vi "fluorescence_timing_pb.vi"(1 "Less frequently changed controls":T2={"Column for Fluorescence"=11, "PB Ch for Blue Image AOM"=5, "PB Ch for Blue MOT AOM"=6, "PB Ch for MOT Shutter"=7, "MOT Shutter Open Time (s)"=0.05}, 2 "Fluorescence Control":T1={"Absorption or Fluorescence?"=0, "MOT flash time (us)"=500.0} {"Absorption or Fluorescence?" items=["Absorption", "Fluorescence"]}, 3 "PulseBlaster Array of Arrays In":T3(array[cluster])=[{"Data Field"=0, "Delay"=0.005, "OP code"=8, "Output Bits"=[FALSE, TRUE, FALSE, FALSE, FALSE, TRUE, FALSE, FALSE, FALSE, FALSE, FALSE, FALSE, FALSE, FALSE, FALSE, FALSE, FALSE, FALSE, FALSE, FALSE, FALSE, FALSE, FALSE, FALSE], "String"="cool mot coils"}, {"Data Field"=300, "Delay"=0.000999, "OP code"=2, "Output Bits"=[FALSE, TRUE, FALSE, FALSE, FALSE, TRUE, FALSE, FALSE, FALSE, FALSE, FALSE, FALSE, FALSE, FALSE, FALSE, FALSE, FALSE, FALSE, FALSE, FALSE, FALSE, FALSE, FALSE, FALSE], "String"="mot load loop"}, {"Data Field"=1, "Delay"=1e-06, "OP code"=3, "Output Bits"=[FALSE, TRUE, FALSE, FALSE, FALSE, TRUE, FALSE, FALSE, FALSE, FALSE, FALSE, FALSE, FALSE, FALSE, FALSE, FALSE, FALSE, FALSE, FALSE, FALSE, FALSE, FALSE, FALSE, FALSE, FALSE], "String"=""}, {"Data Field"=0, "Delay"=0.001, "OP code"=0, "Output Bits"=[FALSE, TRUE, FALSE, FALSE, FALSE, TRUE, TRUE, FALSE, FALSE, FALSE, FALSE, FALSE, FALSE, FALSE, FALSE, FALSE, FALSE, FALSE, FALSE, FALSE, FALSE, FALSE, FALSE, FALSE], "String"=""}, {"Data Field"=2, "Delay"=0.000999, "OP code"=2, "Output Bits"=[FALSE, TRUE, FALSE, FALSE, FALSE, TRUE, TRUE, FALSE, FALSE, FALSE, FALSE, FALSE, FALSE, FALSE, FALSE, FALSE, FALSE, FALSE, FALSE, FALSE, FALSE, FALSE, FALSE, FALSE], "String"="mot decay loop"}, {"Data Field"=4, "Delay"=1e-06, "OP code"=3, "Output Bits"=[FALSE, TRUE, FALSE, FALSE, FALSE, TRUE, TRUE, FALSE, FALSE, FALSE, FALSE, FALSE, FALSE, FALSE, FALSE, FALSE, FALSE, FALSE, FALSE, FALSE, FALSE, FALSE, FALSE, FALSE], "String"=""}, {"Data Field"=0, "Delay"=0.04, "OP code"=0, "Output Bits"=[FALSE, TRUE, FALSE, FALSE, FALSE, TRUE, TRUE, FALSE, FALSE, FALSE, FALSE, FALSE, FALSE, FALSE, FALSE, FALSE, FALSE, FALSE, FALSE, FALSE, FALSE, FALSE, FALSE, FALSE], "String"=""}, {"Data Field"=0, "Delay"=0.00865, "OP code"=0, "Output Bits"=[FALSE, TRUE, FALSE, FALSE, FALSE, FALSE, TRUE, FALSE, FALSE, FALSE, FALSE, FALSE, FALSE, FALSE, FALSE, FALSE, FALSE, FALSE, FALSE, FALSE, FALSE, FALSE, FALSE, FALSE], "String"=""}, {"Data Field"=0, "Delay"=0.004, "OP code"=0, "Output Bits"=[FALSE, TRUE, FALSE, FALSE, FALSE, FALSE, TRUE, FALSE, FALSE, FALSE, FALSE, FALSE, FALSE, FALSE, FALSE, FALSE, FALSE, FALSE, FALSE, FALSE, FALSE, FALSE, FALSE, FALSE], "String"=""}, {"Data Field"=0, "Delay"=0.0045, "OP code"=0, "Output Bits"=[FALSE, TRUE, FALSE, FALSE, FALSE, FALSE, TRUE, FALSE, FALSE, FALSE, FALSE, FALSE, FALSE, FALSE, FALSE, FALSE, FALSE, FALSE, FALSE, FALSE, FALSE, FALSE, FALSE, FALSE], "String"="Blue MOT Cooling Time"}, {"Data Field"=0, "Delay"=5e-05, "OP code"=0, "Output Bits"=[FALSE, TRUE, FALSE, FALSE, FALSE, FALSE, TRUE, FALSE, FALSE, FALSE, FALSE, FALSE, FALSE, FALSE, FALSE, FALSE, FALSE, FALSE, FALSE, FALSE, FALSE, FALSE, FALSE, FALSE], "String"="Red MOT Cooling Time =="}, {"Data Field"=0, "Delay"=0.01, "OP code"=0, "Output Bits"=[FALSE, TRUE, FALSE, FALSE, FALSE, FALSE, TRUE, FALSE, FALSE, FALSE, FALSE, FALSE, FALSE, FALSE, FALSE, FALSE, FALSE, FALSE, FALSE, FALSE, FALSE, FALSE, FALSE, FALSE], "String"="PAS Beam with RED MOT            DELAY TIME BEFORE INTERAC"}, {"Data Field"=0, "Delay"=0.005, "OP code"=0, "Output Bits"=[FALSE, TRUE, FALSE, FALSE, TRUE, FALSE, TRUE, FALSE, FALSE, FALSE, FALSE, FALSE, FALSE, FALSE, FALSE, FALSE, FALSE, FALSE, FALSE, FALSE, FALSE, FALSE, FALSE, FALSE], "String"="image 12 delay (150n=90ndelay) INTERAC TIME"}, {"Data Field"=0, "Delay"=5e-05, "OP code"=0, "Output Bits"=[FALSE, TRUE, FALSE, FALSE, TRUE, FALSE, TRUE, FALSE, FALSE, FALSE, FALSE, FALSE, FALSE, FALSE, FALSE, FALSE, FALSE, FALSE, FALSE, FALSE, FALSE, FALSE, FALSE, FALSE], "String"="image beam on"}, {"Data Field"=0, "Delay"=0.0002, "OP code"=0, "Output Bits"=[FALSE, TRUE, FALSE, FALSE, FALSE, FALSE, TRUE, FALSE, FALSE, FALSE, FALSE, FALSE, FALSE, FALSE, FALSE, FALSE, FALSE, FALSE, FALSE, FALSE, FALSE, FALSE, FALSE, FALSE], "String"="camera minimum exposure time"}, {"Data Field"=0, "Delay"=0.07, "OP code"=0, "Output Bits"=[FALSE, TRUE, FALSE, FALSE, FALSE, FALSE, TRUE, FALSE, FALSE, FALSE, FALSE, FALSE, FALSE, FALSE, FALSE, FALSE, FALSE, FALSE, FALSE, FALSE, FALSE, FALSE, FALSE, FALSE], "String"="PixelFly Readout 1"}, {"Data Field"=0, "Delay"=0.005, "OP code"=0, "Output Bits"=[FALSE, TRUE, FALSE, FALSE, TRUE, FALSE, TRUE, FALSE, FALSE, FALSE, FALSE, FALSE, FALSE, FALSE, FALSE, FALSE, FALSE, FALSE, FALSE, FALSE, FALSE, FALSE, FALSE, FALSE], "String"="shutter opening time"}, {"Data Field"=0, "Delay"=0.0002, "OP code"=0, "Output Bits"=[FALSE, TRUE, FALSE, FALSE, FALSE, FALSE, TRUE, FALSE, FALSE, FALSE, FALSE, FALSE, FALSE, FALSE, FALSE, FALSE, FALSE, FALSE, FALSE, FALSE, FALSE, FALSE, FALSE, FALSE], "String"="Pixelfly exposure 2"}, {"Data Field"=0, "Delay"=0.07, "OP code"=0, "Output Bits"=[FALSE, TRUE, FALSE, FALSE, FALSE, FALSE, TRUE, FALSE, FALSE, FALSE, FALSE, FALSE, FALSE, FALSE, FALSE, FALSE, FALSE, FALSE, FALSE, FALSE, FALSE, FALSE, FALSE, FALSE], "String"="PixelFly readout 2"}, {"Data Field"=0, "Delay"=0.001, "OP code"=6, "Output Bits"=[FALSE, TRUE, FALSE, FALSE, FALSE, FALSE, TRUE, FALSE, FALSE, FALSE, FALSE, FALSE, FALSE, FALSE, FALSE, FALSE, FALSE, FALSE, FALSE, FALSE, FALSE, FALSE, FALSE, FALSE], "String"=""}] {"OP code" items=["Continue", "Stop", "Loop", "End Loop", "Jump", "Return", "Go To", "Long Delay", "Wait"]; "Delay" format="%.3p"}) -> (0 "PB Array of Arrays Out":T3(array[cluster]) {"OP code" items=["Continue", "Stop", "Loop", "End Loop", "Jump", "Return", "Go To", "Long Delay", "Wait"]; "Delay" format="%.2p"})   [LabVIEW 2013]
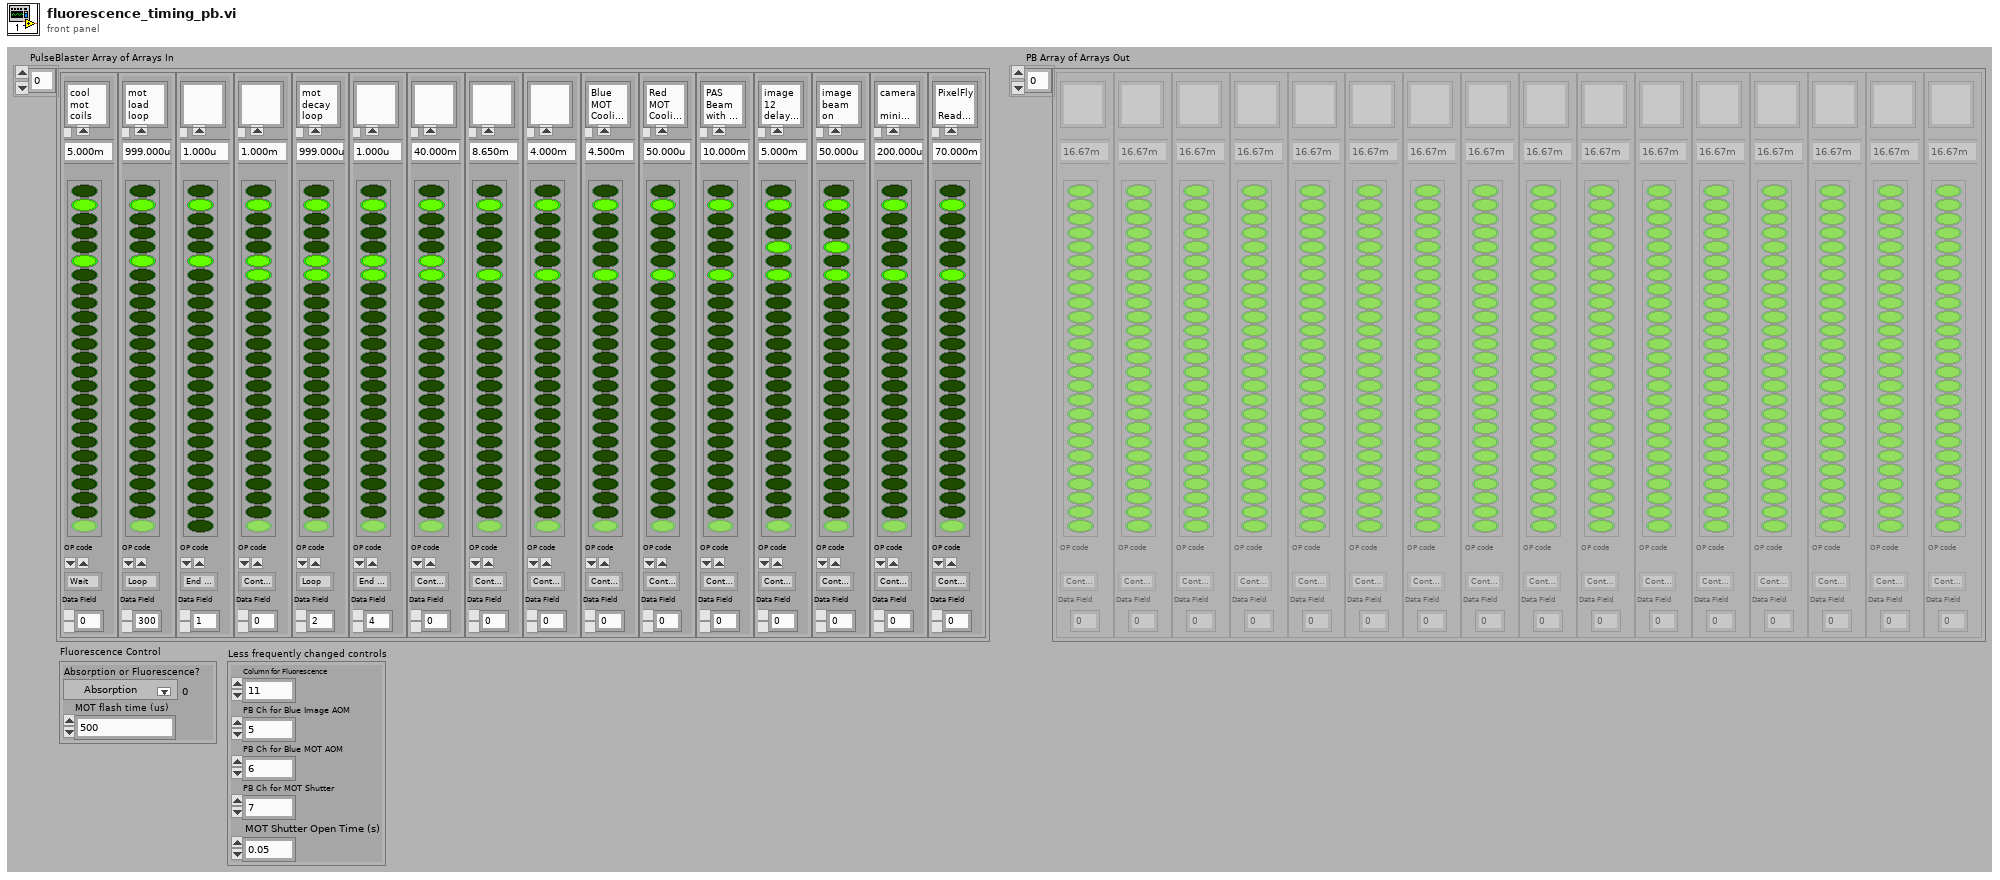
[diagram p1: front panel]
types:
  T1 = cluster{"Absorption or Fluorescence?":u16, "MOT flash time (us)":dbl}
  T2 = cluster{"Column for Fluorescence":i32, "PB Ch for Blue Image AOM":i32, "PB Ch for Blue MOT AOM":i32, "PB Ch for MOT Shutter":i32, "MOT Shutter Open Time (s)":dbl}
  T3 = cluster{"Data Field":u32, "Delay":dbl, "OP code":u8, "Output Bits":bool[], "String":string}[]
  T4 = cluster{"Data Field":u32, "Delay":dbl, "OP code":u8, "Output Bits":bool[], "String":string}
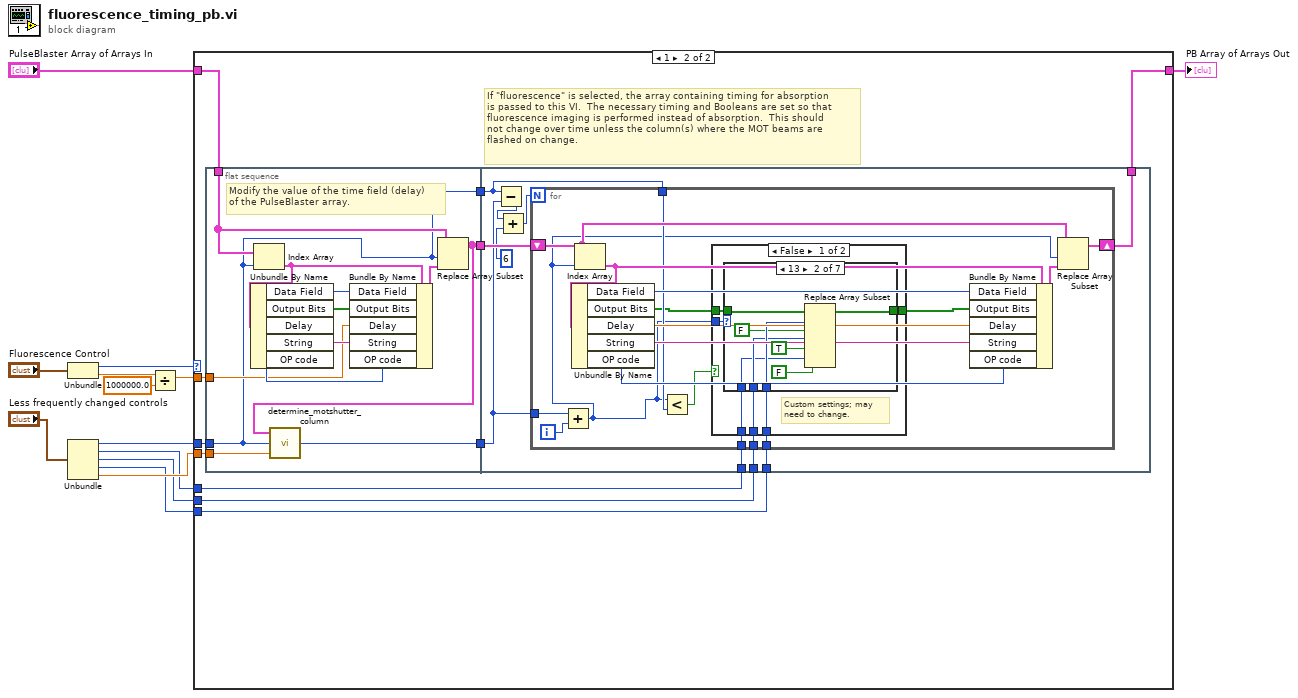
[diagram p0: block diagram]
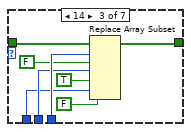
[diagram p4: hidden frame]
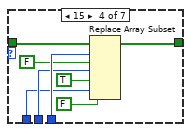
[diagram p5: hidden frame]
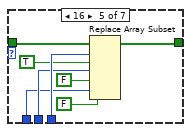
[diagram p6: hidden frame]
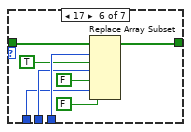
[diagram p7: hidden frame]
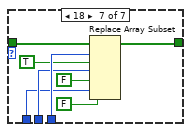
[diagram p8: hidden frame]
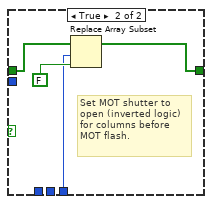
[diagram p9: hidden frame]
diagram:
  n1 = Unbundle("Fluorescence Control") -> ("Absorption or Fluorescence?"=w11:u16, "MOT flash time (us)"=w2:dbl)
  n2 = Unbundle("Less frequently changed controls") -> ("Column for Fluorescence"=w9:i32, "PB Ch for Blue Image AOM"=w6:i32, "PB Ch for Blue MOT AOM"=w5:i32, "PB Ch for MOT Shutter"=w4:i32, "MOT Shutter Open Time (s)"=w7:dbl)
  n3 = Divide(x=w2, y=1000000.0) -> (x/y=w3:dbl)
  n4 = case shown="1" w11 {
    tunnel: "PulseBlaster Array of Arrays In" -> [w14 w25]
    tunnel: w3 -> [_ w24]
    tunnel: w9 -> [_ w23]
    tunnel: [w14 w22] -> w8
    tunnel: w7 -> [_ w19]
    tunnel: w6 -> [_ w17]
    tunnel: w5 -> [_ w16]
    tunnel: w4 -> [_ w15]
    frame 0, Default {
      # "Default is absorption imaging.  The timing on the front panel\nof the PB stays just as it is."
    }
    frame 1 {
      # "If \"fluorescence\" is selected, the array containing timing for absorption\nis passed to this VI.  The necessary timing and Booleans are set so that\nfluorescence imaging is performed instead of absorption.  This should\nnot change over time unless the column(s) where the MOT beams are \nflashed on change."
      n5 = flat-sequence {
        tunnel: w25 -> [w31]
        tunnel: w24 -> [w30]
        tunnel: w23 -> [w26]
        tunnel: [w29] -> w21
        tunnel: [w27] -> w20
        tunnel: w19 -> [w28]
        tunnel: [w26] -> w18
        tunnel: w21 -> [w47]
        tunnel: w20 -> [w45]
        tunnel: [w46] -> w22
        tunnel: w18 -> [w41]
        tunnel: w17 -> [w40]
        tunnel: w16 -> [w39]
        tunnel: w15 -> [w38]
        frame #0 {
          # "Modify the value of the time field (delay)\nof the PulseBlaster array."
          n6 = Index Array(array=w31, index=w26) -> (element=w32:T4)
          n7 = Unbundle By Name(w32) -> ("Data Field"=w33:u32, "Output Bits"=w35:bool[], "String"=w37:string, "OP code"=w36:u8)  [unwired: 1 out]
          n8 = Bundle By Name(cluster=w32, "Data Field"=w33, "Output Bits"=w35, "Delay"=w30, "String"=w37, "OP code"=w36) -> (w34:T4)
          n9 = Replace Array Subset(array=w31, new element=w34, index=w26) -> (w29:T3)
          n10 = call "determine_motshutter_column.vi"("MOT Shutter\nOpening Time (s)"=w28, "Flash Column"=w26, "PulseBlaster Array of Arrays In"=w29) -> ("Column at which\nto open MOT shutter"=w27:i32)
        }
        frame #1 {
          n11 = Subtract(x=w41, y=w45) -> (x-y=w44:i32)
          n12 = Add(x=w44, y=6) -> (x+y=w42:i32)
          n13 = for {
            N: w42 -> [_]
            tunnel: w45 -> [w57]
            shift-right: [w56] -> w46
            shift-left: w47 -> [w60]
            tunnel: w41 -> [w55]
            tunnel: w40 -> [w52]
            tunnel: w39 -> [w51]
            tunnel: w38 -> [w50]
            i -> [w58]
            n14 = Add(x=w57, y=w58) -> (x+y=w49:i32)
            n15 = Index Array(array=w60, index=w49) -> (element=w61:T4)
            n16 = Unbundle By Name(w61) -> ("Data Field"=w62:u32, "Output Bits"=w53:bool[], "Delay"=w59:dbl, "String"=w65:string, "OP code"=w64:u8)
            n17 = Less?(x=w49, y=w55) -> (x < y?=w54:bool)
            n18 = case shown="False" w54 {
              tunnel: w53 -> [w70 w124]
              tunnel: w52 -> [w66 _]
              tunnel: w51 -> [w67 _]
              tunnel: w50 -> [w69 w122]
              tunnel: w49 -> [w71 _]
              tunnel: [w68 w121] -> w48
              frame False {
                # "Custom settings; may\nneed to change."
                n19 = case shown="13" w71 {
                  tunnel: w70 -> [w72 w80 w88 w96 w104 w112 w120]
                  tunnel: w69 -> [_ w79 w87 w95 w103 w111 w119]
                  tunnel: [w72 w76 w84 w92 w100 w108 w116] -> w68
                  tunnel: w67 -> [_ w78 w86 w94 w102 w110 w118]
                  tunnel: w66 -> [_ w74 w82 w90 w98 w106 w114]
                  frame 0, Default {
                    # "If for some reason stuff\ndoes not work, just pass\nalong what's already\nthere."
                  }
                  frame 13 {
                    n20 = Replace Array Subset(array=w80, new element #1=FALSE ("new element/subarray"), index #1=w79, new element #2=TRUE ("new element/subarray"), index #2=w78, new element #3=FALSE, index #3=w74) -> (w76:bool[])
                  }
                  frame 14 {
                    n21 = Replace Array Subset(array=w88, new element #1=FALSE ("new element/subarray"), index #1=w87, new element #2=TRUE ("new element/subarray"), index #2=w86, new element #3=FALSE, index #3=w82) -> (w84:bool[])
                  }
                  frame 15 {
                    n22 = Replace Array Subset(array=w96, new element #1=FALSE ("new element/subarray"), index #1=w95, new element #2=TRUE ("new element/subarray"), index #2=w94, new element #3=FALSE, index #3=w90) -> (w92:bool[])
                  }
                  frame 16 {
                    n23 = Replace Array Subset(array=w104, new element #1=TRUE ("new element/subarray"), index #1=w103, new element #2=FALSE ("new element/subarray"), index #2=w102, new element #3=FALSE, index #3=w98) -> (w100:bool[])
                  }
                  frame 17 {
                    n24 = Replace Array Subset(array=w112, new element #1=TRUE ("new element/subarray"), index #1=w111, new element #2=FALSE ("new element/subarray"), index #2=w110, new element #3=FALSE, index #3=w106) -> (w108:bool[])
                  }
                  frame 18 {
                    n25 = Replace Array Subset(array=w120, new element #1=TRUE ("new element/subarray"), index #1=w119, new element #2=FALSE ("new element/subarray"), index #2=w118, new element #3=FALSE, index #3=w114) -> (w116:bool[])
                  }
                }
              }
              frame True {
                # "Set MOT shutter to\nopen (inverted logic)\nfor columns before\nMOT flash."
                n26 = Replace Array Subset(array=w124, new element=FALSE ("new element/subarray"), index=w122) -> (w121:bool[])
              }
            }
            n27 = Bundle By Name(cluster=w61, "Data Field"=w62, "Output Bits"=w48, "Delay"=w59, "String"=w65, "OP code"=w64) -> (w63:T4)
            n28 = Replace Array Subset(array=w60, new element=w63, index=w49) -> (w56:T3)
          }
        }
      }
    }
  }
  "PB Array of Arrays Out" <- w8
